vi "Msg - Timing.vi"(0 "Message":T1, 11 "error in (no error)":errorcluster) -> (15 "error out":errorcluster)   [LabVIEW 2016, in "Template.lvlib"]
doc: "Send a Message to this Module to setup its Timer VI"
uses:
  Template.lvlib
  Controls/Timing - Setup.ctl
  Controls/Timing - Mode.ctl
  Controls/Message.ctl
  Controls/Module - States.ctl
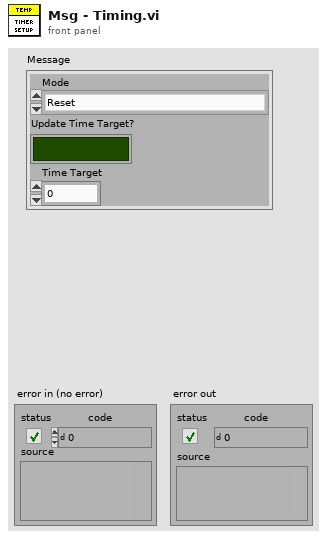
[diagram p1: front panel]
types:
  T1 = typedef "Template.lvlib/Timing - Setup.ctl" = cluster{"Mode":T2, "Update Time Target?":bool, "Time Target":dbl}
  T2 = typedef "Template.lvlib/Timing - Mode.ctl" = enum16{"Reset", "Read", "Pause", "Resume"}
  T3 = typedef "Template.lvlib/Message.ctl" = cluster{"State":T4, "Data":variant, "Transitioning State?":bool}
  T4 = typedef "Template.lvlib/Module - States.ctl" = enum16{"Initialize", "Event ", "Send data", "FP Element: Update", "FP Element: Disable/Enable", "Timer: Setup", "Terminate", "---------------Template---------------"}
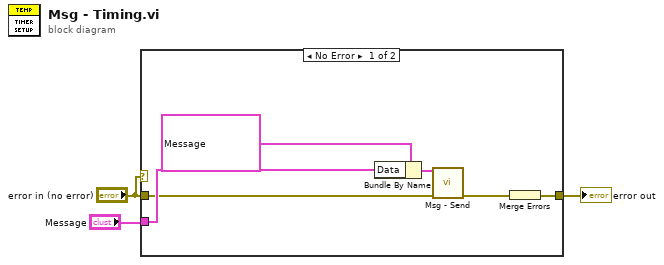
[diagram p0: block diagram]
diagram:
  n1 = case shown="No Error" "error in (no error)" {
    tunnel: [w5 w10] -> w3
    tunnel: "error in (no error)" -> [w7 w10]
    tunnel: "Message" -> [w9 _]
    frame No Error {
      n2 = Bundle By Name(cluster=T3 {"State"=enum."Timer: Setup", "Data"=variant, "Transitioning State?"=FALSE} ("Message"), "Data"=w9) -> (w4:T3)
      n3 = call "Msg - Send.vi"("Message"=w4, "error in (no error)"=w7) -> ("error out"=w6:errorcluster)  [unwired: 13 in]
      n4 = Merge Errors(w6) -> (w5:errorcluster)
    }
    frame Error {
    }
  }
  "error out" <- w3
